vi "Close Window.vi"(0 "Document in":refnum<class "Document.lvclass">, 11 "error in (no error)":errorcluster) -> (4 "Document out":refnum<class "Document.lvclass">, 15 "error out":errorcluster)   [LabVIEW 2016, in "Document.lvclass"]
uses:
  Document.lvclass
  Document.lvclass/Document.ctl
  user32.dll
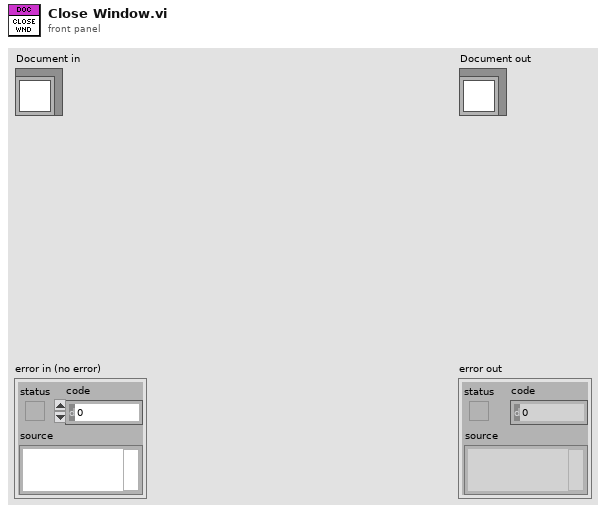
[diagram p1: front panel]
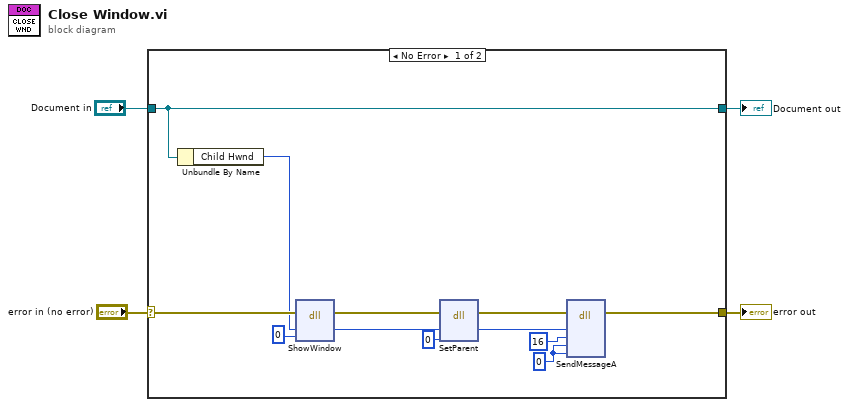
[diagram p0: block diagram]
diagram:
  n1 = case shown="No Error" "error in (no error)" {
    selector: "error in (no error)" -> [w8 w18]
    tunnel: [w7 w18] -> w3
    tunnel: [w6 w17] -> w1
    tunnel: "Document in" -> [w6 w17]
    frame No Error {
      w12 = u32 0 ("wParam")
      n2 = Unbundle By Name(w6) -> ("Child Hwnd"=w5:u32)
      n3 = dll-call lib="user32.dll" fn="ShowWindow"(error in=w8, "hwnd"=w5, "nCmdShow"=u32 0) -> (error out=w10:errorcluster, "hwnd"=w14:u32)  [unwired: 4 in, 1 out]
      n4 = dll-call lib="user32.dll" fn="SetParent"(error in=w10, "Child"=w14, "NewParent"=0) -> (error out=w9:errorcluster, "Child"=w11:u32)  [unwired: 4 in, 1 out]
      n5 = dll-call lib="user32.dll" fn="SendMessageA"(error in=w9, "hwnd"=w11, "msg"=u32 16, "wParam"=w12, "lParam"=w12) -> (error out=w7:errorcluster)  [unwired: 7 in, 1 out]
    }
    frame Error {
    }
  }
  "error out" <- w3
  "Document out" <- w1
